vi "host.vi"() -> ()   [LabVIEW 2020]
uses:
  <vilib>/Analysis/baseanly.llb/Vector x A.vi
  <vilib>/Analysis/baseanly.llb/Real Dot Product.vi
  <vilib>/Analysis/Matrix/Numeric/Conversions/Array To Matrix - RA2.vi
  <vilib>/rvi/interface/RandomDataEmulation/nirviRandomDataOpen.vi
  <vilib>/rvi/interface/common/niFpgaCacheSessionInfoDynamic.vi
  <vilib>/Utility/error.llb/Error Cluster From Error Code.vi
  <vilib>/rvi/errors/niLvFpgaAdjustHostInterfaceError.vi
  <vilib>/FPGAPlugInAG/Dynamic/niLvFpga_Run_Dynamic.vi
  <vilib>/FPGAPlugInAG/Dynamic/niLvFpga_Close_Dynamic.vi
  <vilib>/rvi/interface/nirviOpenFPGA/nirviOpenFPGA.xnode
  target.vi
  <vilib>/rvi/interface/nirviMethod/nirviMethod.xnode
  <vilib>/rvi/interface/nirviReadWriteControl/nirviReadWriteControl.xnode
  <vilib>/rvi/interface/nirviCloseFPGA/nirviCloseFPGA.xnode
  <vilib>/Analysis/NI_AALBase.lvlib
  <vilib>/Analysis/Matrix/NI_Matrix.lvlib
  <vilib>/FPGAPlugInAG/Dynamic/niLvFpga_WriteFifo_Dynamic.vi
  <vilib>/rvi/errors/niLvFpgaMergeErrorWithErrorCode.vi
  NiFpgaLv.dll
  <vilib>/rvi/interface/Simulation/niFpgaSimulationCallBeginRW.vi
panel:
  out "clock ticks":u32
  out "error":dbl
  out "y (CPU)":dbl
  out "y (FPGA)":fxp<+/-,33,17>
  out "subarray":fxp<+/-,32,16>[](array[numeric])
  out "V' x A 2":dbl[](array[numeric])
  out "Waveform Graph":waveform(dbl)(graph)
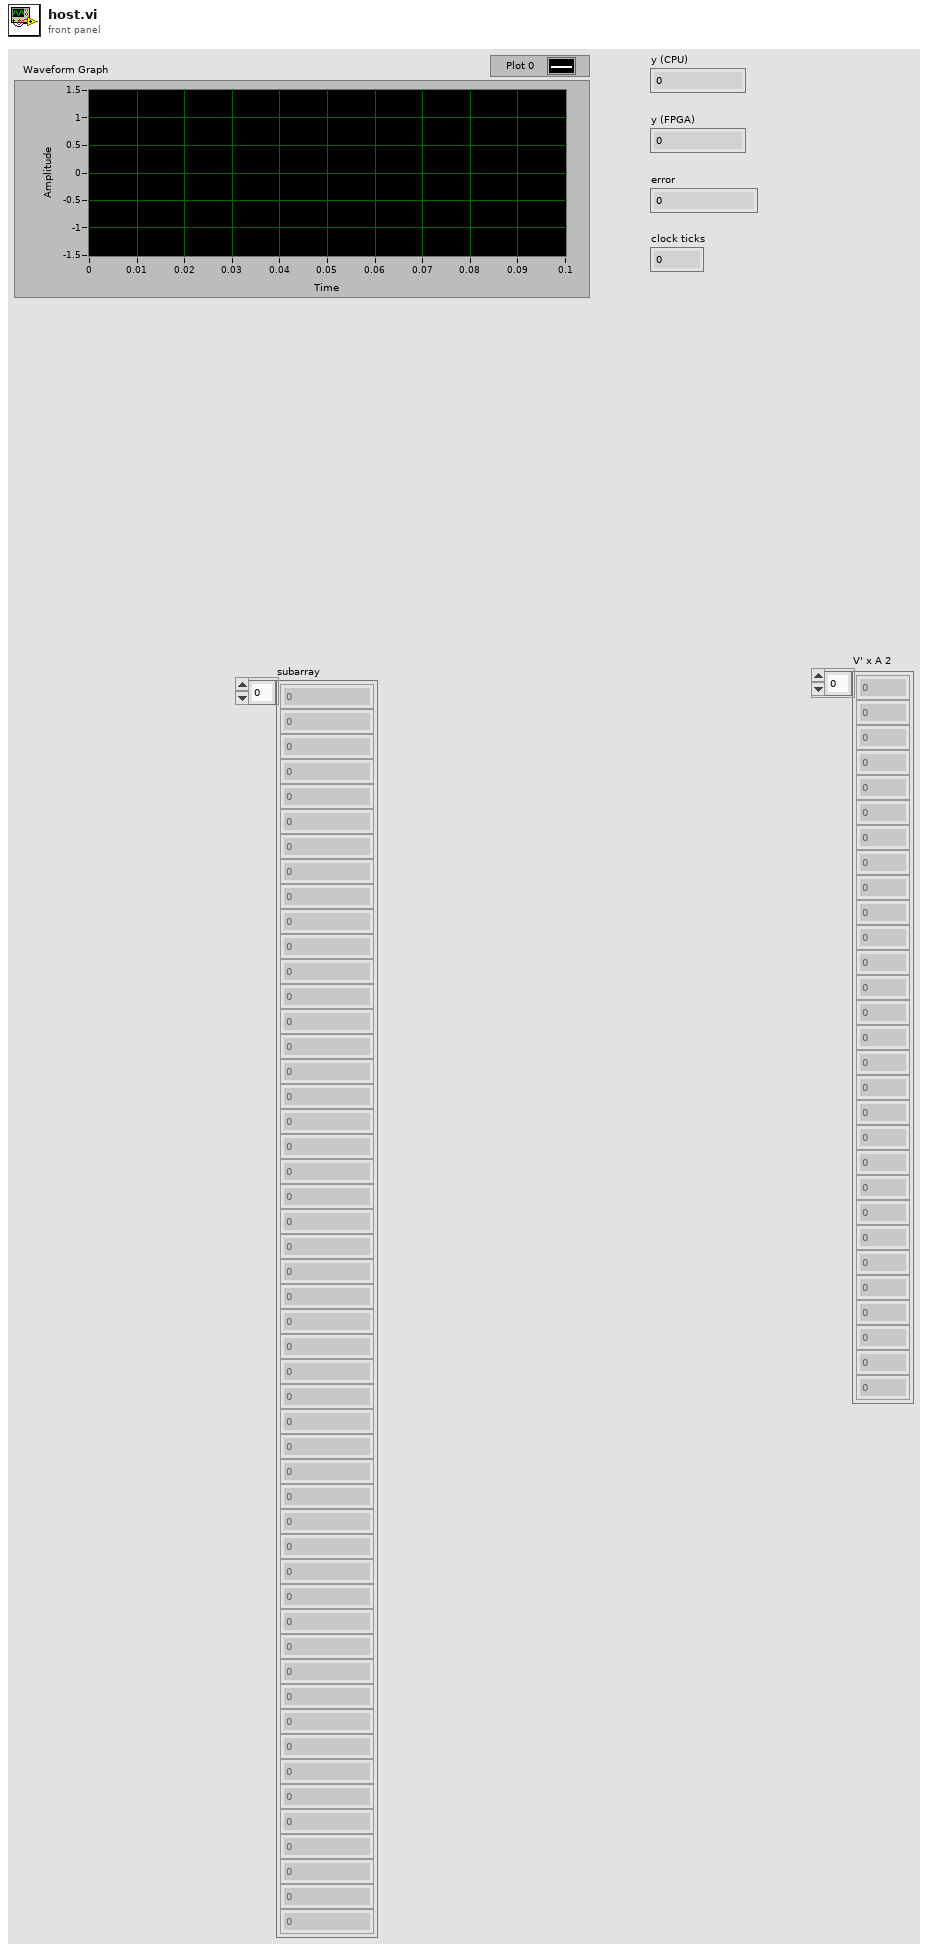
[diagram p1: front panel]
types:
  T1 = typedef "NI_Matrix.lvlib/RealMatrix.ctl" = dbl[][]
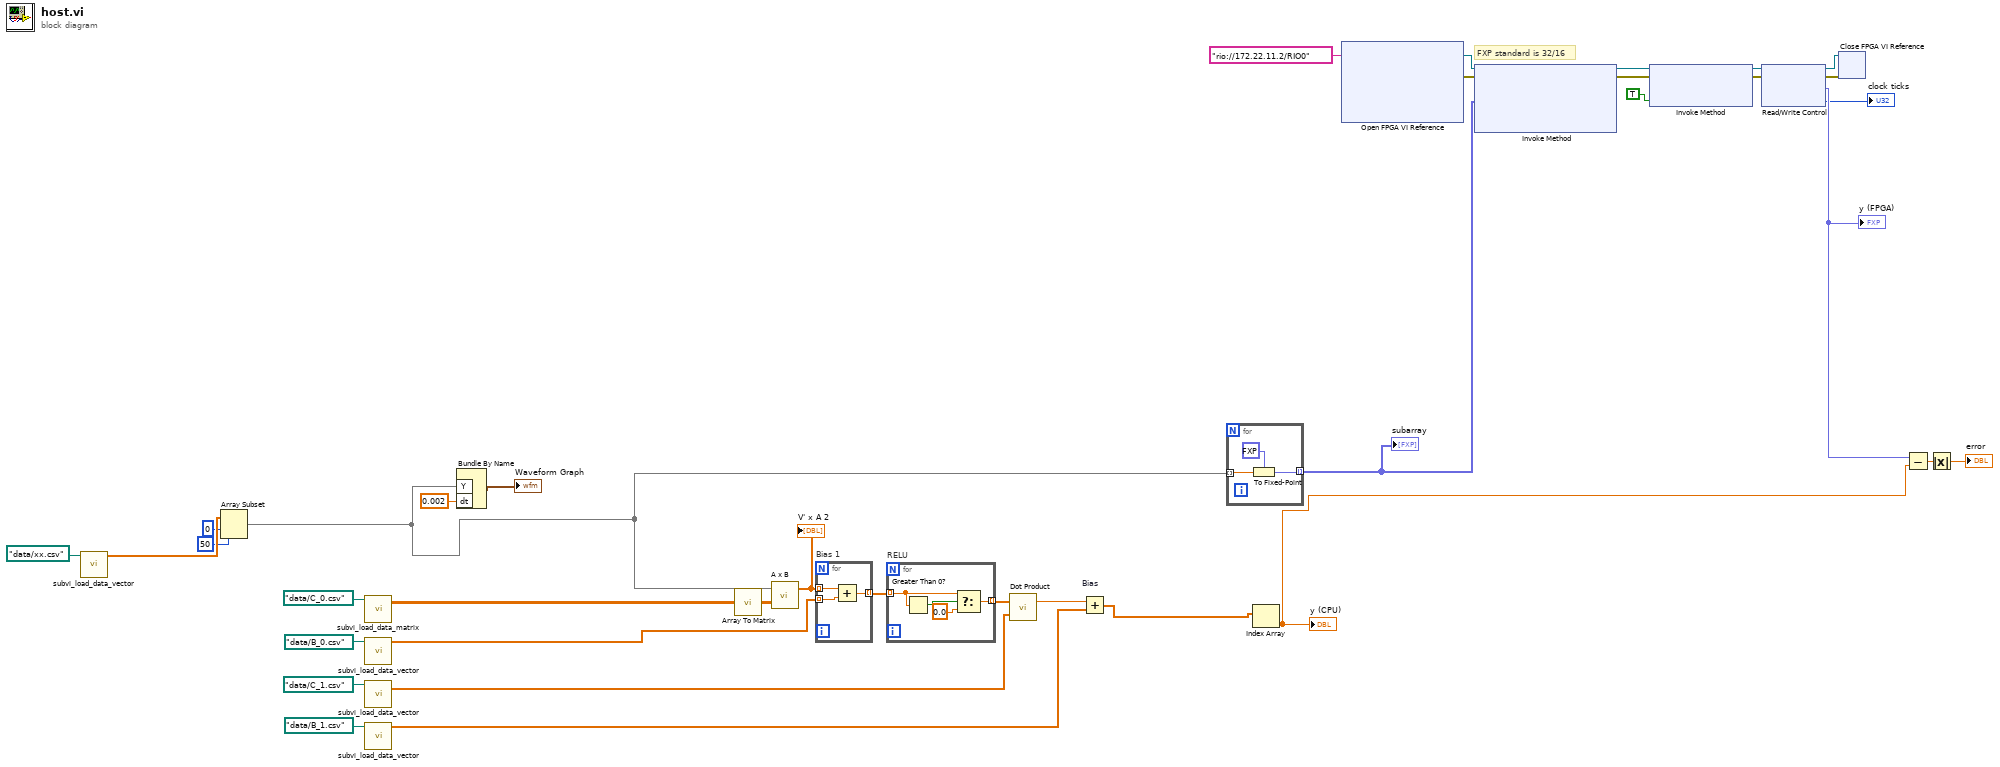
[diagram p0: block diagram]
diagram:
  # "FXP standard is 32/16"
  n1 = call "subvi_load_data_vector.vi"("default name"=path "data/xx.csv") -> ("array type (2D Dbl) out"=w10:dbl[])  [unwired: 10 in]
  n2 = Array Subset(array=w10, index=0, length=50) -> (w9:dbl[])
  n3 = call "subvi_load_data_matrix.vi"("default name"=path "data/C_0.csv") -> ("array"=w23:dbl[][])  [unwired: 10 in]
  n4 = call "subvi_load_data_vector.vi"("default name"=path "data/B_0.csv") -> ("array type (2D Dbl) out"=w22:dbl[])  [unwired: 10 in]
  n5 = call "subvi_load_data_vector.vi"("default name"=path "data/C_1.csv") -> ("array type (2D Dbl) out"=w19:dbl[])  [unwired: 10 in]
  n6 = call "subvi_load_data_vector.vi"("default name"=path "data/B_1.csv") -> ("array type (2D Dbl) out"=w21:dbl[])  [unwired: 10 in]
  n7 = Bundle By Name("Y"=w9, "dt"=0.002) -> (→"Waveform Graph":waveform(dbl))  [unwired: 1 in]
  n8 = call-poly <vilib>:"Array To Matrix.vi"("Real 2D Array"=w23) -> ("Real Matrix"=w16:T1)
  n9 = call-poly <vilib>:"A x B.vi"("Matrix A"=w16, "Vector V'"=w9) -> ("V' x A"=w31:dbl[])  [unwired: 1 out]
  "V' x A 2" <- w31
  n10 = for "Bias 1" {
    tunnel: w31 -> [w40] mode=indexing
    tunnel: [w39] -> w30 mode=indexing
    tunnel: w22 -> [w38] mode=indexing
    n11 = Add(x=w40, y=w38) -> (x+y=w39:dbl)
  }
  n12 = for "RELU" {
    tunnel: w30 -> [w44] mode=indexing
    tunnel: [w43] -> w20 mode=indexing
    n13 = Greater Than 0?(x=w44) -> (x > 0?=w41:bool)
    n14 = Select(t=w44, s=w41, f=0.0) -> (s? t:f=w43:dbl)
  }
  n15 = call-poly <vilib>:"Dot Product.vi"("Y Vector"=w19, "X Vector"=w20) -> ("X * Y"=w29:dbl)  [unwired: 1 out]
  n16 = Add "Bias"(x=w29, y=w21) -> (x+y=w4:dbl[])
  n17 = for {
    tunnel: w9 -> [w46] mode=indexing
    tunnel: [w45] -> w15 mode=indexing
    n18 = To Fixed-Point(fixed-point type=fxp<+/-,32,16> 0.0 ("fixed-point"), number=w46) -> (fixed-point=w45:fxp<+/-,32,16>)
  }
  "subarray" <- w15
  n19 = Index Array(array=w4) -> (element=w3:dbl)  [unwired: 1 in]
  "y (CPU)" <- w3
  n20 = xnode "Open FPGA VI Reference"("resource name"=tag "rio://172.22.11.2/RIO0") -> ("FPGA VI Reference Out"=w37:refnum<k20>, "error out"=w36:errorcluster)  [unwired: 1 in]
  n21 = xnode "Invoke Method"("FPGA VI Reference In"=w37, "error in"=w36, "Data"=w15) -> ("FPGA VI Reference Out"=w18:refnum<k20>, "error out"=w17:errorcluster)  [unwired: 1 in, 1 out]
  n22 = xnode "Invoke Method"("FPGA VI Reference In"=w18, "error in"=w17, "Wait Until Done (F)"=TRUE) -> ("FPGA VI Reference Out"=w14:refnum<k20>, "error out"=w13:errorcluster)
  n23 = xnode "Read/Write Control"("FPGA VI Reference In"=w14, "error in"=w13) -> ("FPGA VI Reference Out"=w12:refnum<k20>, "error out"=w11:errorcluster, "y"=w5:fxp<+/-,33,17>, "clock ticks"=→"clock ticks":u32)
  "y (FPGA)" <- w5
  n24 = xnode "Close FPGA VI Reference"("FPGA VI Reference In"=w12, "error in"=w11) -> ()  [unwired: 1 out]
  n25 = Subtract(x=w5, y=w3) -> (x-y=w6:dbl)
  n26 = Absolute Value(x=w6) -> (abs(x)=→"error":dbl)
